vi "move convert to conti.vi"(9 "Position":T3, 10 "path array":T4[](array[typedef])) -> (0 "VAJ path":T1[](array[typedef]), 2 "path":T2[](array[typedef]))   [LabVIEW 2019]
uses:
  ctl/path ctl.ctl
  ctl/position name.ctl
  subVI/move/position cluster.ctl
  subVI/move control/move and align/move_cluster.ctl
  subVI/move control/move and align/V A J control/move cluster(VAJ).ctl
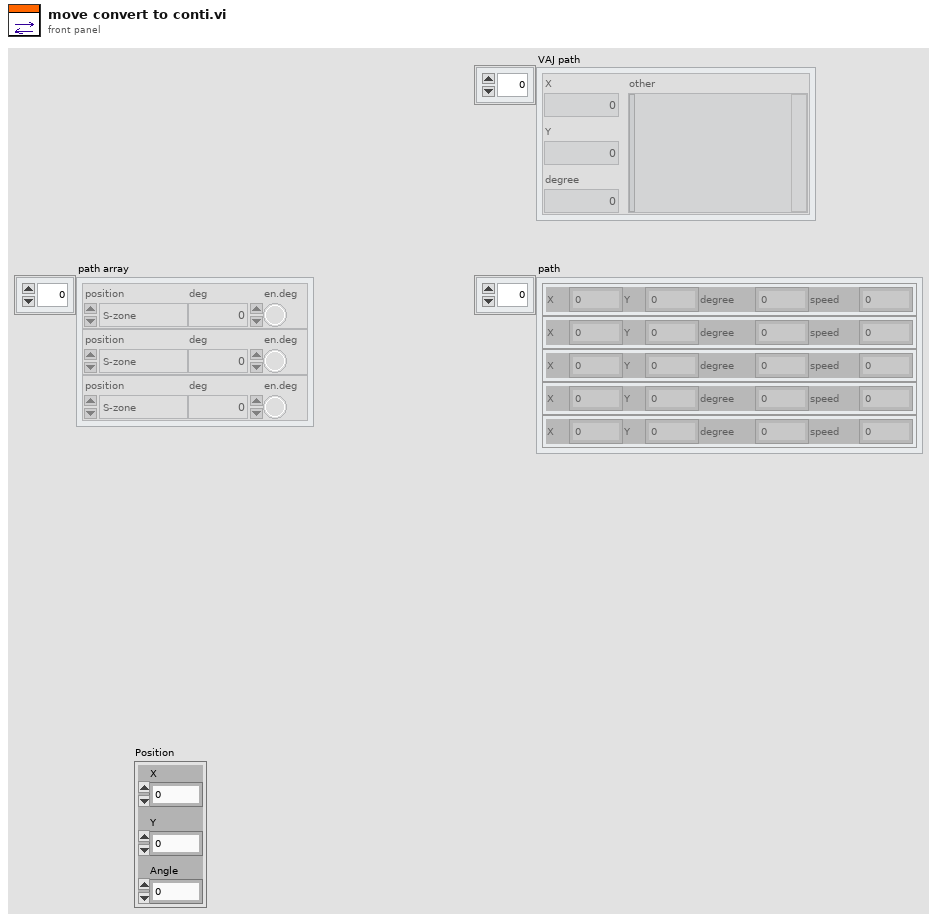
[diagram p1: front panel]
types:
  T1 = typedef "move cluster(VAJ).ctl" = cluster{"X":dbl, "Y":dbl, "degree":dbl, "other":string}
  T2 = typedef "move_cluster.ctl" = cluster{"X":dbl, "Y":dbl, "degree":dbl, "speed":dbl}
  T3 = typedef "position cluster.ctl" = cluster{"X":dbl, "Y":dbl, "Angle":dbl}
  T4 = typedef "path ctl.ctl" = cluster{"position":T5, "deg":dbl, "en.deg":bool}
  T5 = typedef "position name.ctl" = enum16{"S-zone", "out S", "vision board-vision", "out box", "box catch", "room center", "room right", "room left", "R2", "R4", "only rotate", "out recy", "recycle", "R3", "near board", "box poxition", "R1", "R5", "R1-d", "R5-d", "R3.4", "align center.1", "align center.5", "R2-d", "R2-r", "far center"}
  T6 = typedef "position array.ctl" = cluster{"position":T5, "X":dbl, "Y":dbl}
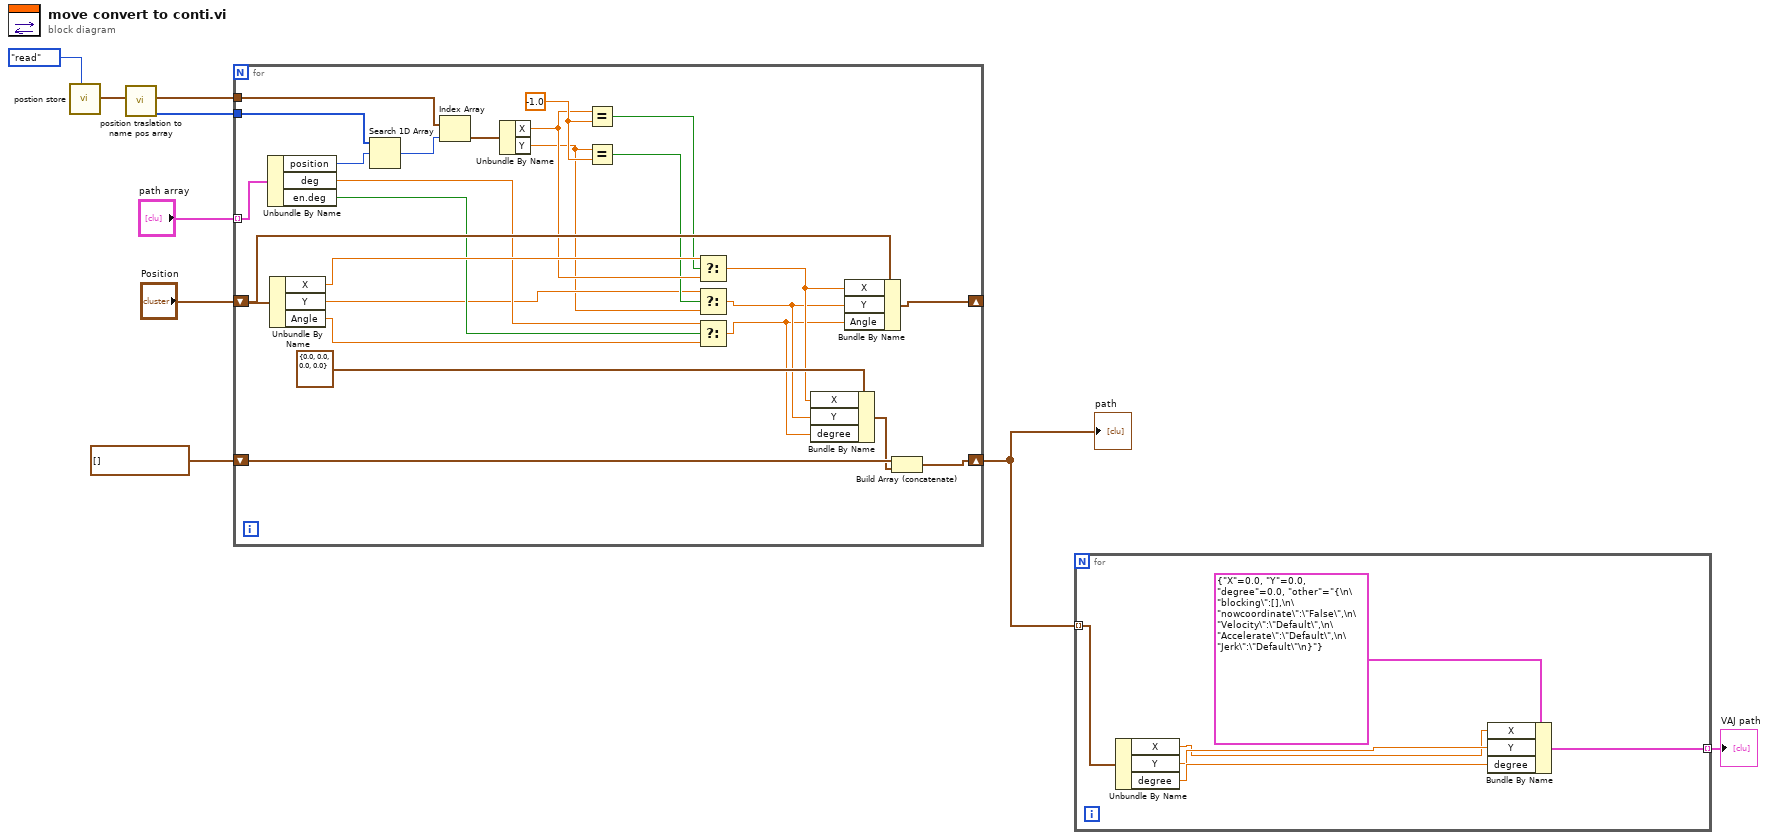
[diagram p0: block diagram]
diagram:
  n1 = call "postion store.vi"("R/W"=enum16{"write", "read"}."read") -> ("read"=w5:T6[])  [unwired: 10 in]
  n2 = call "position traslation to name pos array.vi"("Array"=w5) -> ("name array"=w3:T5[], "pos array"=w4:cluster{"X":dbl, "Y":dbl}[])  [unwired: 9 in]
  n3 = for {
    tunnel: "path array" -> [w32] mode=indexing
    shift-right: [w10] -> w2
    shift-left: T2[] [] ("Array") -> [w34]
    shift-right: [w24] -> _
    shift-left: "Position" -> [w25]
    tunnel: w4 -> [w28]
    tunnel: w3 -> [w30]
    w23 = -1.0 ("y")
    n4 = Unbundle By Name(w32) -> ("position"=w31:T5, "deg"=w16:dbl, "en.deg"=w17:bool)
    n5 = Unbundle By Name(w25) -> ("X"=w22:dbl, "Y"=w14:dbl, "Angle"=w15:dbl)
    n6 = Search 1D Array(1D array=w30, element=w31) -> (index of element=w29:i32)  [unwired: 1 in]
    n7 = Index Array(array=w28, index=w29) -> (element=w26:cluster{"X":dbl, "Y":dbl})
    n8 = Unbundle By Name(w26) -> ("X"=w21:dbl, "Y"=w13:dbl)
    n9 = Equal?(x=w21, y=w23) -> (x = y?=w19:bool)
    n10 = Equal?(x=w13, y=w23) -> (x = y?=w18:bool)
    n11 = Select(t=w22, s=w19, f=w21) -> (s? t:f=w20:dbl)
    n12 = Select(t=w14, s=w18, f=w13) -> (s? t:f=w12:dbl)
    n13 = Select(t=w16, s=w17, f=w15) -> (s? t:f=w11:dbl)
    n14 = Bundle By Name(cluster=T2 {"X"=0.0, "Y"=0.0, "degree"=0.0, "speed"=0.0} ("Cluster"), "X"=w20, "Y"=w12, "degree"=w11) -> (w27:T2)
    n15 = Bundle By Name(cluster=w25, "X"=w20, "Y"=w12, "Angle"=w11) -> (w24:T3)
    n16 = Build Array (concatenate)(w34, w27) -> (w10:T2[])
  }
  "path" <- w2
  n17 = for {
    tunnel: w2 -> [w39] mode=indexing
    tunnel: [w35] -> w1 mode=indexing
    n18 = Unbundle By Name(w39) -> ("X"=w36:dbl, "Y"=w37:dbl, "degree"=w38:dbl)
    n19 = Bundle By Name(cluster=T1 {"X"=0.0, "Y"=0.0, "degree"=0.0, "other"="{\n\"blocking\":[],\n\"nowcoordinate\":\"False\",\n\"Velocity\":\"Default\",\n\"Accelerate\":\"Default\",\n\"Jerk\":\"Default\"\n}"} ("move in"), "X"=w36, "Y"=w37, "degree"=w38) -> (w35:T1)
  }
  "VAJ path" <- w1
